vi "SR430_reset.vi"(0 "address":T1, 5 "error in (no error)":errorcluster) -> (14 "address out":T1, 19 "error out":errorcluster={"status"=TRUE, "code"=6, "source"="GPIB Write in SR430_reset.vi"})   [LabVIEW 2009, in "SR430Driver.lvlib"]
doc: "Clears all status register, sends a \"device clear\" and resets the SR430 to its default configuration.\n\nCopyright (C)\nGesellschaft für Schwerionenforschung, GSI\nPlanckstr. 1\n64291 Darmstadt\nGermany\n\nContact: D.Beck@gsi.de \n\nThis program is free software; you can redistribute it and/or modify it under the terms of the \nGNU General Public License as published by the Free Software Foundation; either version 2 of the license, or (at your option) any later version.\n\nThis program is distributed in the hope that it will be useful, but WITHOUT ANY WARRANTY; without even the implied warranty of MERCHANTABILITY or FITNESS FOR A PARTICULAR PURPOSE. See the GNU General License for more details (http://www.gnu.org).\n\nGesellschaft für Schwerionenforschung, GSI\nPlanckstr. 1, 64291 Darmstadt, Germany\nFor all questions and ideas contact: M.Richter@gsi.de, K.Poppensieker, H.Brand@gsi.de or D.Beck@gsi.de.\nLast update: 11-APR-2002"
uses:
  SR430Driver.lvlib
  SR430_VISA Control.ctl
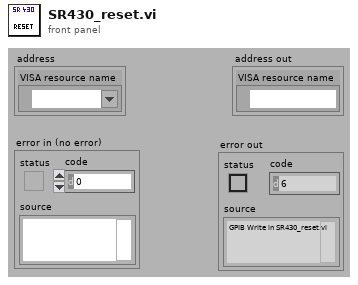
[diagram p1: front panel]
types:
  T1 = typedef "SR430Driver.lvlib/SR430_VISA Control.ctl" = cluster{"VISA resource name":refnum<visa-resource-name>}
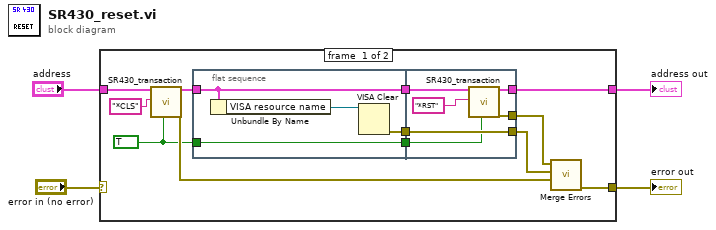
[diagram p0: block diagram]
diagram:
  n1 = case shown="No Error" "error in (no error)" {
    selector: "error in (no error)" -> [_ w28]
    tunnel: [w11 w28] -> w3
    tunnel: "address" -> [w16 w27]
    tunnel: [w14 w27] -> w1
    frame #0 {
      w6 = TRUE
      n2 = call "SR430_transaction.vi"("SR430 VISA Cluster"=w16, "SR430 Command String"="*CLS", "ignoreInterfaceReady (FALSE)"=w6) -> ("dup SR430 VISA Cluster"=w12:T1, "error out"=w7:errorcluster)  [unwired: 13 in, 2 out]
      n3 = flat-sequence {
        tunnel: [w19] -> w13
        tunnel: w12 -> [w19]
        tunnel: [w18] -> w8
        tunnel: w6 -> [w17]
        tunnel: [w17] -> w5
        tunnel: [w25] -> w14
        tunnel: w13 -> [w24]
        tunnel: [w23] -> w10
        tunnel: [w22] -> w9
        tunnel: w8 -> [w22]
        tunnel: w5 -> [w21]
        frame #0 {
          n4 = Unbundle By Name(w19) -> ("VISA resource name"=w20:refnum<visa-resource-name>)
          n5 = VISA Clear(VISA resource name=w20) -> (error out=w18:errorcluster)  [unwired: 1 in, 1 out]
        }
        frame #1 {
          n6 = call "SR430_transaction.vi"("SR430 VISA Cluster"=w24, "SR430 Command String"="*RST" ("data"), "ignoreInterfaceReady (FALSE)"=w21) -> ("dup SR430 VISA Cluster"=w25:T1, "error out"=w23:errorcluster)  [unwired: 13 in, 2 out]
        }
      }
      n7 = call <vilib>:"Merge Errors.vi"("error in 3 (no error)"=w7, "error in 2 (no error)"=w9, "error in 1 (no error)"=w10) -> ("error out"=w11:errorcluster)  [unwired: 4 in]
    }
    frame #1 {
    }
  }
  "error out" <- w3
  "address out" <- w1
